vi "motor safety.vi"(1 "no signal cutoff rate":dbl=0.2, 2 "Motor Output":dbl, 3 "Current Rate":dbl) -> (0 "Safe Motor Output":dbl)   [LabVIEW 2011]
uses:
  fg_typedef.ctl
  DB DataType Custom.ctl
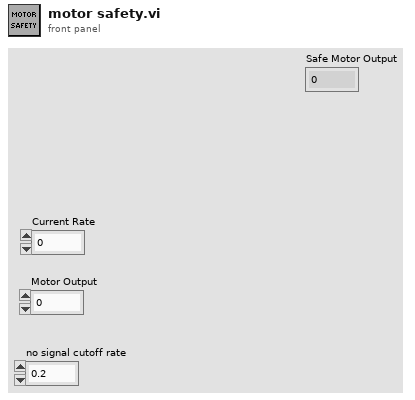
[diagram p1: front panel]
types:
  T1 = typedef "DB DataType Custom.ctl" = enum16{"VLAD Balanced", "Turret Safety", "Turret Limit"}
  T2 = typedef "fg_typedef.ctl" = enum16{"Get", "Set"}
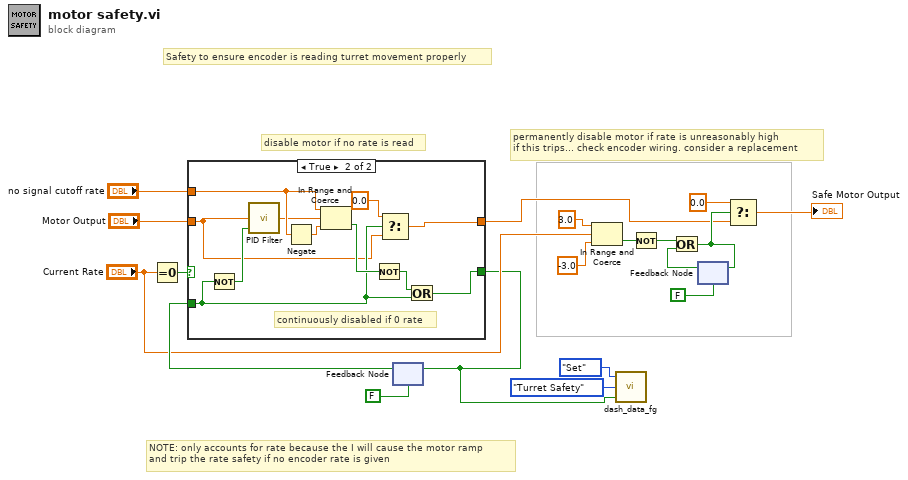
[diagram p0: block diagram]
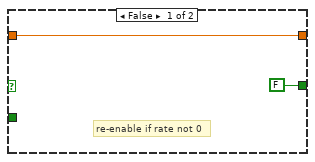
[diagram p2: hidden frame]
diagram:
  # "Safety to ensure encoder is reading turret movement properly"
  # "NOTE: only accounts for rate because the I will cause the motor ramp\nand trip the rate safety if no encoder rate is given"
  # "permanently disable motor if rate is unreasonably high\nif this trips... check encoder wiring. consider a replacement"
  # "disable motor if no rate is read"
  n1 = Equal To 0?(x="Current Rate") -> (x = 0?=w18:bool)
  n2 = feedback #1(FALSE ("x > y?")) -> (w11:bool)
  n3 = case shown="True" w18 {
    tunnel: "Motor Output" -> [w21 w23]
    tunnel: [w21 w31] -> w5
    tunnel: [FALSE w28] -> w1
    tunnel: w11 -> [_ w27]
    tunnel: "no signal cutoff rate" -> [_ w25]
    frame False {
      # "re-enable if rate not 0"
    }
    frame True {
      # "continuously disabled if 0 rate"
      n4 = Not(x=w27) -> (.not. x?=w24:bool)
      n5 = call "PID Filter.vi"("reinitialize? (F)"=w24, "input"=w23) -> ("output"=w22:dbl)  [unwired: 3 in]
      n6 = Negate(x=w25) -> (-x=w26:dbl)
      n7 = In Range and Coerce(upper limit=w25, x=w22, lower limit=w26) -> (In Range?=w30:bool)  [unwired: 1 out]
      n8 = Not(x=w30) -> (.not. x?=w29:bool)
      n9 = Select(t=0.0, s=w27, f=w23) -> (s? t:f=w31:dbl)
      n10 = Or(x=w29, y=w27) -> (x .or. y?=w28:bool)
    }
  }
  n11 = feedback-in #1(w1) -> ()
  n12 = In Range and Coerce(upper limit=3.0 ("y"), x="Current Rate", lower limit=-3.0 ("y")) -> (In Range?=w7:bool)  [unwired: 1 out]
  n13 = call "dash_data_fg.vi"("Input"=w1, "DB DataType"=DB_DataType_Custom."Turret Safety", "Menu (Get)"=fg_typedef."Set") -> ()  [unwired: 1 out]
  n14 = Not(x=w7) -> (.not. x?=w6:bool)
  n15 = feedback #2(FALSE ("x > y?")) -> (w15:bool)
  n16 = Or(x=w6, y=w15) -> (x .or. y?=w14:bool)
  n17 = feedback-in #2(w14) -> ()
  n18 = Select(t=0.0, s=w14, f=w5) -> (s? t:f=→"Safe Motor Output":dbl)
